vi "CNR abx reweighted.vi"(0 "parameters":dbl[](array[numeric]), 1 "model function":T4, 5 "method":T2 items=["Least Square", "Least Absolute Residual", "Bisquare"], 7 "scale factors":dbl[](array[numeric]), 9 "output control":T3={"model function"=TRUE, "gradient"=TRUE}, 11 "error in (no error)":errorcluster, 12 "Y":dbl[](array[numeric]), 13 "X":dbl[](array[numeric]), 14 "Weight":dbl[](array[numeric])) -> (2 "Jacobian":T1, 3 "number of function calls":i32, 4 "Hessian":T1, 6 "gradient":dbl[](array[numeric]), 8 "best fit":dbl[](array[numeric]), 10 "chiSqr":dbl, 15 "error out":errorcluster)   [LabVIEW 2010, in "NI_Gmath.lvlib"]
uses:
  NI_Gmath.lvlib
  RealMatrix.ctl
  LM model function.ctl
  LM model function reference.ctl
  LM_output select.ctl
  Curve Fitting Criteria.ctl
  Real Dot Product.vi
  Real A x B.vi
  A x Vector.vi
  NI_AALBase.lvlib
  NI_Matrix.lvlib
  NI_AALPro.lvlib
panel:
  # "Lev-Mar\nabx"
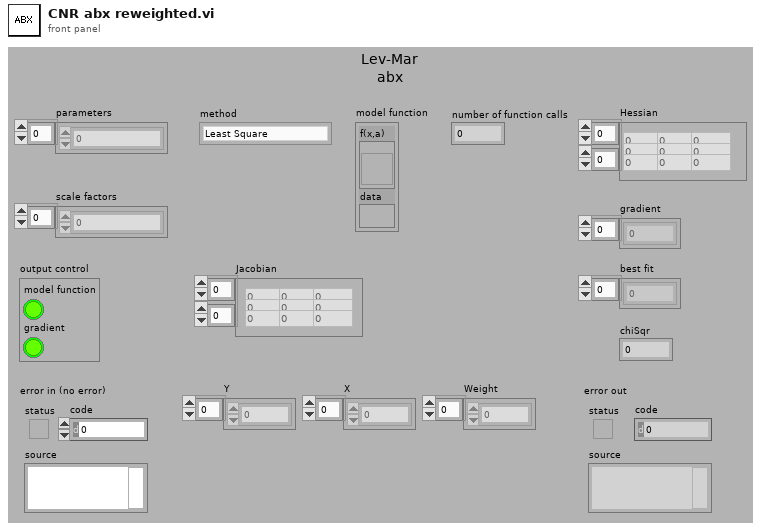
[diagram p1: front panel]
types:
  T1 = typedef "NI_Matrix.lvlib/RealMatrix.ctl" = dbl[][]
  T2 = typedef "NI_AALPro.lvlib/Curve Fitting Criteria.ctl" = u16
  T3 = typedef "NI_Gmath.lvlib/LM_output select.ctl" = cluster{"model function":bool, "gradient":bool}
  T4 = typedef "NI_Gmath.lvlib/LM model function.ctl" = cluster{"f(x,a)":T5, "data":variant}
  T5 = typedef "NI_Gmath.lvlib/LM model function reference.ctl" = refnum<vi>
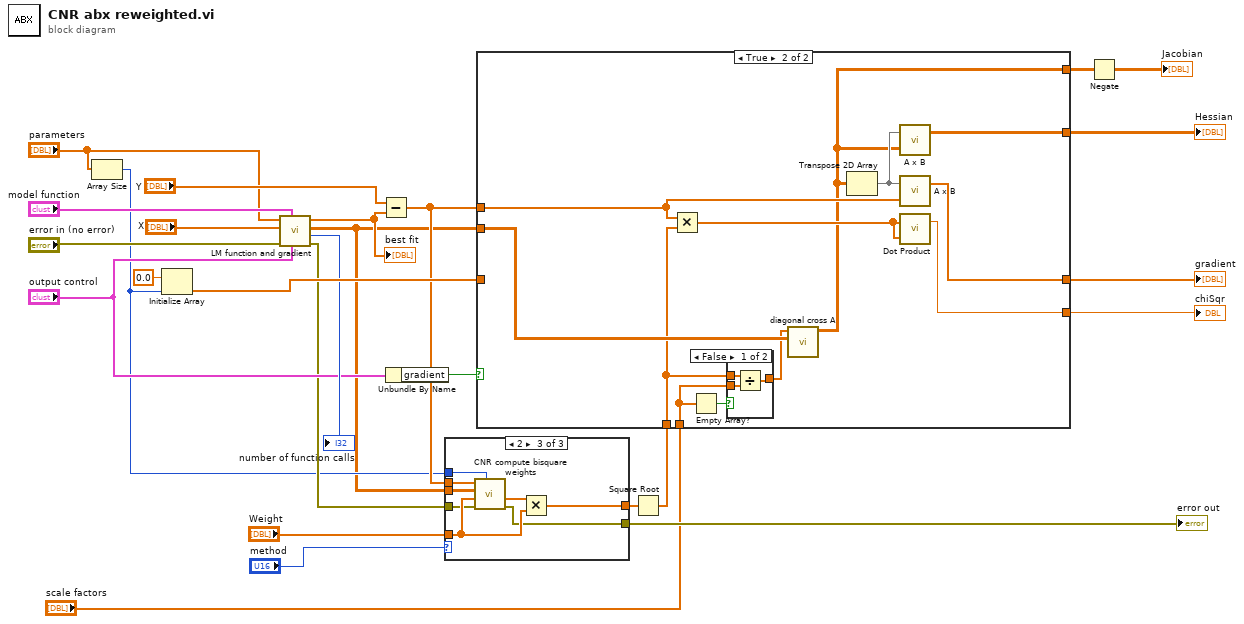
[diagram p0: block diagram]
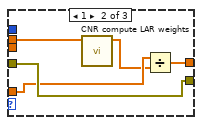
[diagram p3: hidden frame]
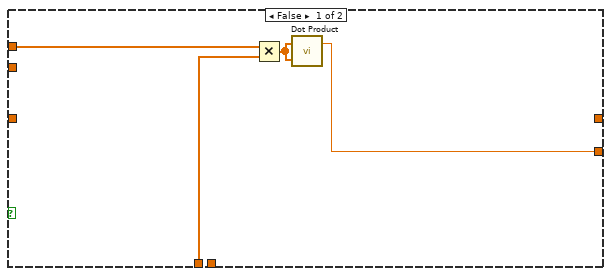
[diagram p4: hidden frame]
diagram:
  n1 = Array Size(array="parameters") -> (size(s)=w8:i32)
  n2 = Initialize Array(0.0, w8) -> (w25:dbl[])
  n3 = call "LM function and gradient.vi"("output control"="output control", "model function"="model function", "error in (no error)"="error in (no error)", "X"="X", "a"="parameters") -> ("error out"=w16:errorcluster, "number of function calls"=→"number of function calls":i32, "gradient"=w3:dbl[][], "f(X)"=w18:dbl[])  [unwired: 3 out]
  "best fit" <- w18
  n4 = Subtract(x="Y", y=w18) -> (x-y=w9:dbl[])
  n5 = Unbundle By Name("output control") -> ("gradient"=w20:bool)
  n6 = case shown="2" "method" {
    tunnel: w3 -> [_ _ w41]
    tunnel: [w28 w31 w40] -> w5
    tunnel: "Weight" -> [w28 w32 w39]
    tunnel: [w27 w33 w38] -> w12
    tunnel: w16 -> [w27 w33 w37]
    tunnel: w9 -> [_ w30 w36]
    tunnel: w8 -> [_ _ w34]
    frame 0, Default {
    }
    frame 1 {
      n7 = call "CNR compute LAR weights.vi"("residuals"=w30) -> ("LAR weights"=w29:dbl[])  [unwired: 10 out]
      n8 = Divide(x=w32, y=w29) -> (x/y=w31:dbl[])
    }
    frame 2 {
      n9 = call "CNR compute bisquare weights.vi"("number of parameters"=w34, "error in (no error)"=w37, "weight"=w39, "J"=w41, "raw residuals"=w36) -> ("error out"=w38:errorcluster, "weights"=w35:dbl[])  [unwired: 5 out]
      n10 = Multiply(x=w35, y=w39) -> (x*y=w40:dbl[])
    }
  }
  "error out" <- w12
  n11 = Square Root(x=w5) -> (sqrt(x)=w6:dbl[])
  n12 = case shown="True" w20 {
    tunnel: w25 -> [_ _]
    tunnel: [_ w46] -> w13
    tunnel: [_ w47] -> w1
    tunnel: [w42 w57] -> w24
    tunnel: w3 -> [_ w56]
    tunnel: w6 -> [w45 w52]
    tunnel: w9 -> [w44 w55]
    tunnel: "scale factors" -> [_ w50]
    tunnel: [_ w48] -> w2
    frame False {
      n13 = Multiply(x=w44, y=w45) -> (x*y=w43:dbl[])
      n14 = call-poly "Dot Product.vi"("Y Vector"=w43, "X Vector"=w43) -> ("X * Y"=w42:dbl)  [unwired: 1 out]
    }
    frame True {
      n15 = Multiply(x=w55, y=w52) -> (x*y=w53:dbl[])
      n16 = Empty Array?(array=w50) -> (empty?=w49:bool)
      n17 = case shown="False" w49 {
        tunnel: w52 -> [w60 w61]
        tunnel: w50 -> [w59 _]
        tunnel: [w58 w61] -> w51
        frame False {
          n18 = Divide(x=w60, y=w59) -> (x/y=w58:dbl[])
        }
        frame True {
        }
      }
      n19 = call "diagonal cross A.vi"("A"=w56, "diagonal"=w51) -> ("diagonalxA"=w48:T1)  [unwired: 9 out]
      n20 = Transpose 2D Array(2D array=w48) -> (transposed array=w54:T1)
      n21 = call-poly "A x B.vi"("B"=w48, "A"=w54) -> ("A x B"=w47:T1)  [unwired: 1 out]
      n22 = call-poly "A x B.vi"("Vector"=w55, "A"=w54) -> ("A x Vector"=w46:dbl[])  [unwired: 1 out]
      n23 = call-poly "Dot Product.vi"("Y Vector"=w53, "X Vector"=w53) -> ("X * Y"=w57:dbl)  [unwired: 1 out]
    }
  }
  "Hessian" <- w1
  "gradient" <- w13
  "chiSqr" <- w24
  n24 = Negate(x=w2) -> (-x=→"Jacobian":T1)
